vi "Basic ReadWrite.vi"() -> ()   [LabVIEW 2020]
doc: "This is an example using the VIT Super Network Streams class for reading and writing withing the same application.\n\nCopyright © 2008 - 2024 VI Technologies B.V. \nALL RIGHTS RESERVED"
uses:
  SuperNS/SuperNS.lvclass
  MsgData/MsgData.lvclass
panel:
  out "Received":string
  in  "Send":bool
  in  "Msg":string
  in  "ShowWin":bool
  # "Copyright (c) 2024, VI Technologies B.V.\nAll rights reserved.\n\nRedistribution and use in source and binary forms, with or without modification, are permitted provided that \nthe following conditions are met:\n\n * Redistributions of source code must retain the above copyright notice, this list of conditions and the \nfollowing disclaimer.\n * Redistributions in binary form must reproduce the above copyright notice, this list of conditions and the \nfollowing disclaimer in the documentation and/or other materials provided with the distribution.\n * Neither the name of VI Technologies B.V. nor the names of its contributors may be used to endorse or \npromote products derived from this software without specific prior written permission.\n\nTHIS SOFTWARE IS PROVIDED BY THE COPYRIGHT HOLDERS AND CONTRIBUTORS \"AS IS\" AND ANY EXPRESS OR \nIMPLIED WARRANTIES, INCLUDING, BUT NOT LIMITED TO, THE IMPLIED WARRANTIES OF MERCHANTABILITY \nAND FITNESS FOR A PARTICULAR PURPOSE ARE DISCLAIMED. IN NO EVENT SHALL THE COPYRIGHT OWNER OR \nCONTRIBUTORS BE LIABLE FOR ANY DIRECT, INDIRECT, INCIDENTAL, SPECIAL, EXEMPLARY, OR CONSEQUENTIAL \nDAMAGES (INCLUDING, BUT NOT LIMITED TO, PROCUREMENT OF SUBSTITUTE GOODS OR SERVICES; LOSS OF \nUSE, DATA, OR PROFITS; OR BUSINESS INTERRUPTION) HOWEVER CAUSED AND ON ANY THEORY OF LIABILITY, \nWHETHER IN CONTRACT, STRICT LIABILITY, OR TORT (INCLUDING NEGLIGENCE OR OTHERWISE) ARISING IN ANY \nWAY OUT OF THE USE OF THIS SOFTWARE, EVEN IF ADVISED OF THE POSSIBILITY OF SUCH DAMAGE.\n\nFor more information, please visit https://www.vi-tech.nl or contact us at info@vi-tech.nl"
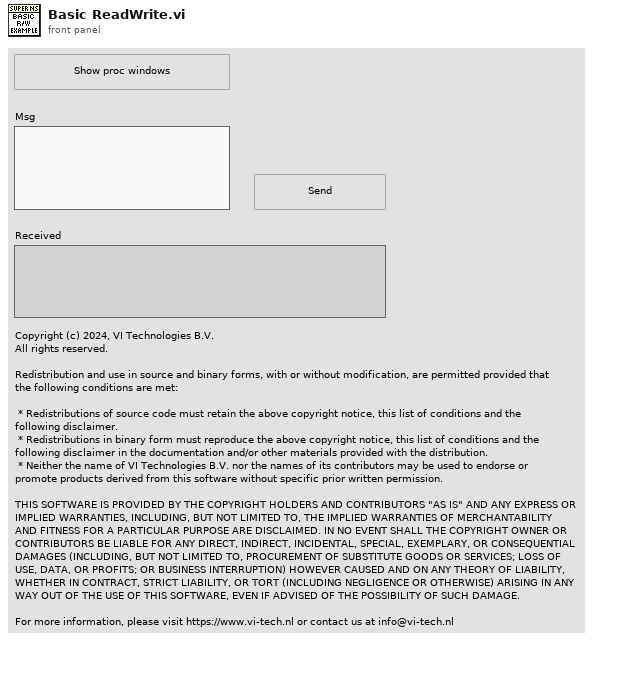
[diagram p1: front panel]
types:
  T1 = typedef "SuperNS.lvclass/StreamDataType.ctl" = refnum<class>
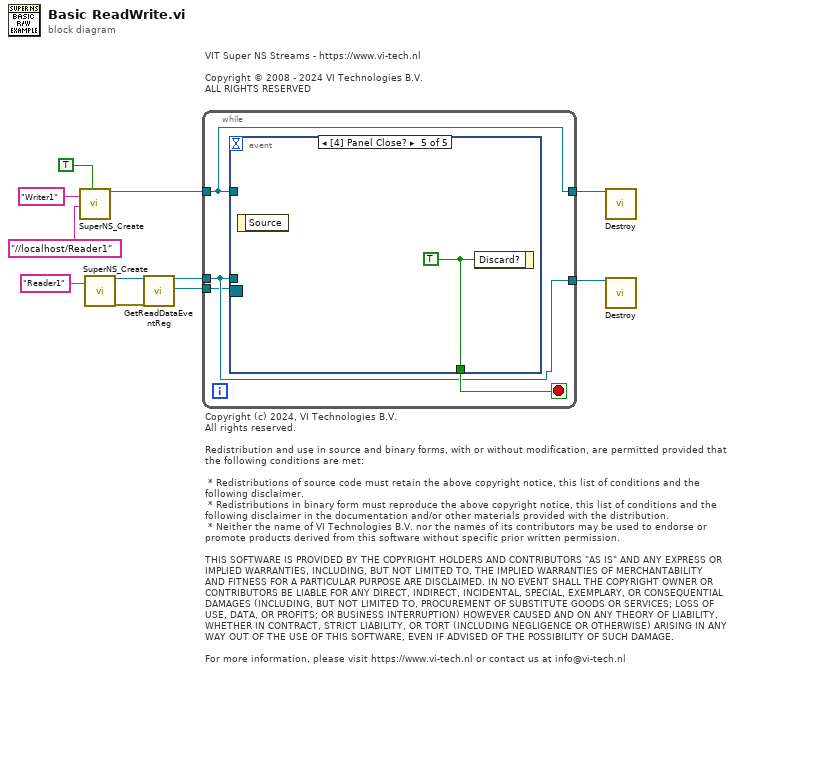
[diagram p0: block diagram]
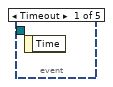
[diagram p2: hidden frame]
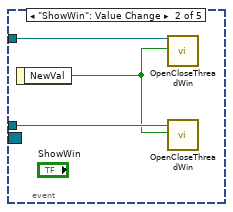
[diagram p3: hidden frame]
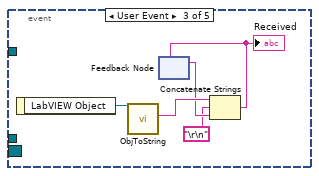
[diagram p4: hidden frame]
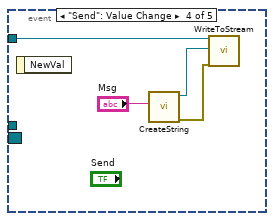
[diagram p5: hidden frame]
diagram:
  # "VIT Super NS Streams - https://www.vi-tech.nl\n\nCopyright © 2008 - 2024 VI Technologies B.V. \nALL RIGHTS RESERVED"
  # "Copyright (c) 2024, VI Technologies B.V.\nAll rights reserved.\n\nRedistribution and use in source and binary forms, with or without modification, are permitted provided that \nthe following conditions are met:\n\n * Redistributions of source code must retain the above copyright notice, this list of conditions and the \nfollowing disclaimer.\n * Redistributions in binary form must reproduce the above copyright notice, this list of conditions and the \nfollowing disclaimer in the documentation and/or other materials provided with the distribution.\n * Neither the name of VI Technologies B.V. nor the names of its contributors may be used to endorse or \npromote products derived from this software without specific prior written permission.\n\nTHIS SOFTWARE IS PROVIDED BY THE COPYRIGHT HOLDERS AND CONTRIBUTORS \"AS IS\" AND ANY EXPRESS OR \nIMPLIED WARRANTIES, INCLUDING, BUT NOT LIMITED TO, THE IMPLIED WARRANTIES OF MERCHANTABILITY \nAND FITNESS FOR A PARTICULAR PURPOSE ARE DISCLAIMED. IN NO EVENT SHALL THE COPYRIGHT OWNER OR \nCONTRIBUTORS BE LIABLE FOR ANY DIRECT, INDIRECT, INCIDENTAL, SPECIAL, EXEMPLARY, OR CONSEQUENTIAL \nDAMAGES (INCLUDING, BUT NOT LIMITED TO, PROCUREMENT OF SUBSTITUTE GOODS OR SERVICES; LOSS OF \nUSE, DATA, OR PROFITS; OR BUSINESS INTERRUPTION) HOWEVER CAUSED AND ON ANY THEORY OF LIABILITY, \nWHETHER IN CONTRACT, STRICT LIABILITY, OR TORT (INCLUDING NEGLIGENCE OR OTHERWISE) ARISING IN ANY \nWAY OUT OF THE USE OF THIS SOFTWARE, EVEN IF ADVISED OF THE POSSIBILITY OF SUCH DAMAGE.\n\nFor more information, please visit https://www.vi-tech.nl or contact us at info@vi-tech.nl"
  n1 = call "SuperNS_Create.vi"("NSName"="Writer1", "RemoteEP_URL"="//localhost/Reader1", "Writer (F: Reader)"=TRUE ("Writer")) -> ("SuperNS Reference"=w11:refnum<class "SuperNS.lvclass">)  [unwired: 15 in, 1 out]
  n2 = call "SuperNS_Create.vi"("NSName"="Reader1") -> ("SuperNS Reference"=w8:refnum<class "SuperNS.lvclass">, "error out"=w1:errorcluster)  [unwired: 17 in]
  n3 = call-dynamic "GetReadDataEventReg.vi"("reference in"=w8, "error in"=w1) -> ("reference out"=w3:refnum<class "SuperNS.lvclass">, "SuperNS ReadData"=w2:refnum<event-registration>)  [unwired: 15 in, 1 out]
  n4 = while {
    tunnel: w11 -> [w14]
    tunnel: [w14] -> w10
    tunnel: w3 -> [w13]
    tunnel: [w13] -> w7
    tunnel: w2 -> [w12]
    stop <- w15 stop-if-true
    n5 = event shown="[4] Panel Close?" {
      selector: w12 -> [_ _ _ _ _]
      dyn-events: _ -> [_ _ _ _ _]
      timeout: _ -> [_ _ _ _ _]
      tunnel: [_ _ _ _ w28] -> w15
      tunnel: w14 -> [_ w18 _ w26 _]
      tunnel: w13 -> [_ w17 _ _ _]
      event Timeout {
        n6 = event-data() -> ()  [unwired: 1 in, 1 out]
      }
      event "ShowWin": Value Change {
        n7 = event-data() -> ("NewVal"=w16:bool)  [unwired: 1 in]
        n8 = call-dynamic "OpenCloseThreadWin.vi"("reference in"=w18, "Open (F: Close)"=w16) -> ()  [unwired: 16 in, 2 out]
        n9 = call-dynamic "OpenCloseThreadWin.vi"("reference in"=w17, "Open (F: Close)"=w16) -> ()  [unwired: 16 in, 2 out]
      }
      event User Event {
        n10 = event-data() -> ("LabVIEW Object"=w23:T1)  [unwired: 1 in]
        n11 = call "ObjToString.vi"("LabVIEW Object"=w23) -> ("String"=w22:string)  [unwired: 9 in, 1 out]
        n12 = feedback #1() -> (w20:string)  [unwired: 1 in]
        n13 = Concatenate Strings(w22, "\r\n", w20) -> (w21:string)
        "Received" <- w21
        n14 = feedback-in #1(w21) -> ()
      }
      event "Send": Value Change {
        n15 = event-data() -> ()  [unwired: 1 in, 1 out]
        n16 = call "CreateString.vi"("String"="Msg") -> ("error out"=w24:errorcluster, "MsgData out"=w25:refnum<class "MsgData.lvclass">)  [unwired: 9 in]
        n17 = call-dynamic "WriteToStream.vi"("reference in"=w26, "LabVIEW Object"=w25, "error in"=w24) -> ()  [unwired: 14 in, 3 out]
      }
      event Panel Close? {
        w28 = TRUE ("Discard?")
        n18 = event-data() -> ()  [unwired: 1 in, 1 out]
        n19 = event-data("Discard?"=w28) -> ()  [unwired: 1 in, 1 out]
      }
    }
  }
  n20 = call-dynamic "Destroy.vi"("reference in"=w10) -> ()  [unwired: 17 in, 2 out]
  n21 = call-dynamic "Destroy.vi"("reference in"=w7) -> ()  [unwired: 17 in, 2 out]
